vi "autointerpreter.vi"(1 "String":string="0,5,3,1") -> (0 "Array":T1[](array[typedef]))   [LabVIEW 2012, in "MainProject.lvrbt"]
uses:
  MainProject.lvrbt
  Drivers/AutoControl3.ctl
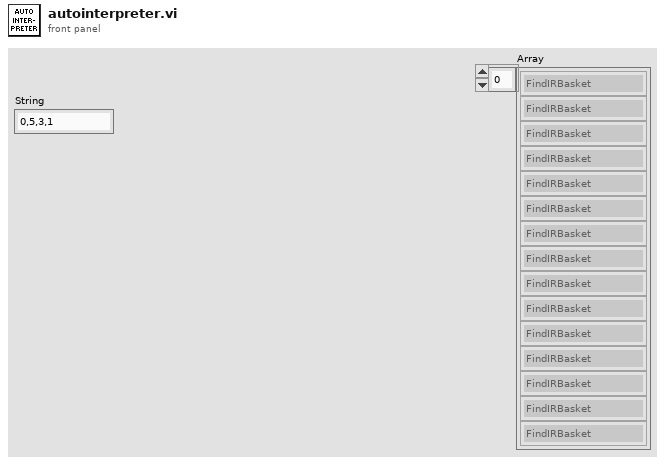
[diagram p1: front panel]
types:
  T1 = typedef "AutoControl3.ctl" = enum16{"FindIRBasket", "DropBLK", "DrvToEndOfBaskets", "DrvAroundBaskets", "AlignWithRamp", "ParkOnRamp", "Stop"}
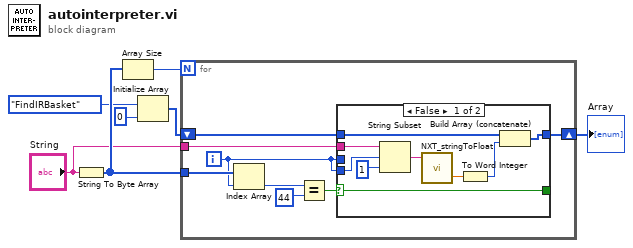
[diagram p0: block diagram]
diagram:
  n1 = String To Byte Array(string="String") -> (unsigned byte array=w7:u8[])
  n2 = Array Size(array=w7) -> (size(s)=w5:i32)
  n3 = Initialize Array(AutoControl3."FindIRBasket" ("Enum"), 0 ("dimension size")) -> (w4:T1[])
  n4 = for {
    N: w5 -> [_]
    tunnel: w7 -> [w11]
    shift-right: [w9] -> w1
    shift-left: w4 -> [w12]
    tunnel: "String" -> [w10]
    i -> [w8]
    n5 = Index Array(array=w11, index=w8) -> (element=w13:u8)
    n6 = Equal?(x=w13, y=u8 44) -> (x = y?=w14:bool)
    n7 = case shown="False" w14 {
      selector: w14 -> [w24 w26]
      tunnel: [w24 w26] -> _
      tunnel: w8 -> [_ _]
      tunnel: w12 -> [w19 w25]
      tunnel: [w17 w25] -> w9
      tunnel: w10 -> [w23 _]
      tunnel: w8 -> [w22 _]
      frame False {
        n8 = String Subset(string=w23, offset (0)=w22, length (rest)=1 ("length (rest)")) -> (substring=w20:string)
        n9 = call <vilib>:"NXT_stringToFloat.vi"("string"=w20) -> ("number"=w18:sgl)  [unwired: 2 in, 1 out]
        n10 = To Word Integer(number=w18) -> (16bit integer=w16:i16)
        n11 = Build Array (concatenate)(w19, w16) -> (w17:u16[])
      }
      frame True {
      }
    }
  }
  "Array" <- w1
